vi "Plot Current_BU.vi"(7 "Current Mode":u8[](array[numeric]), 10 "plot setting":refnum<vi>) -> ()   [LabVIEW 2023]
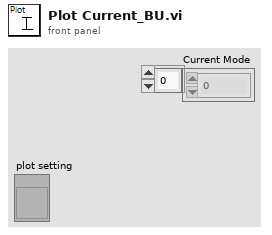
[diagram p1: front panel]
types:
  T1 = cluster{"V plot":bool, "I plot":bool, "Plot colour":u32, "Channel name\n":string}[]
  T2 = cluster{"V plot":bool, "I plot":bool, "Plot colour":u32, "Channel name\n":string}
  T3 = cluster{bool, "I plot":bool, "Plot colour":u32, "Channel name\n":string}
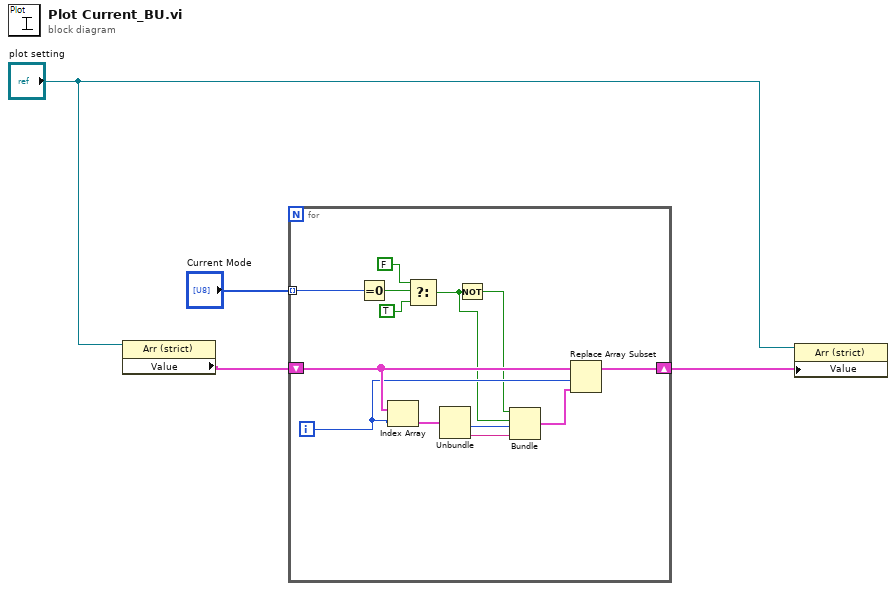
[diagram p0: block diagram]
diagram:
  n1 = property class="Arr (strict)"(reference="plot setting") -> ("Value"=w2:T1)  [unwired: 1 in, 2 out]
  n2 = for {
    tunnel: "Current Mode" -> [w17] mode=indexing
    shift-right: [w5] -> w3
    shift-left: w2 -> [w13]
    i -> [w12]
    n3 = Equal To 0?(x=w17) -> (x = 0?=w16:bool)
    n4 = Index Array(array=w13, index=w12) -> (element=w11:T2)
    n5 = Select(t=FALSE ("I plot"), s=w16, f=TRUE ("I plot")) -> (s? t:f=w7:bool)
    n6 = Unbundle(w11) -> ("Plot colour"=w10:u32, "Channel name"=w9:string)  [unwired: 2 out]
    n7 = Not(x=w7) -> (.not. x?=w8:bool)
    n8 = Bundle(w8, "I plot"=w7, "Plot colour"=w10, "Channel name"=w9) -> (w6:T3)  [unwired: 1 in]
    n9 = Replace Array Subset(array=w13, new element=w6, index=w12) -> (w5:T1)
  }
  n10 = property class="Arr (strict)"(reference="plot setting", "Value"=w3) -> ()  [unwired: 1 in, 2 out]
